vi "GET_sendStatusToClient.vi"() -> (0 "position":dbl, 1 "mode":string)   [LabVIEW 2024]
uses:
  <vilib>/wsapi/Web Request.lvclass
  Main.vi
panel:
  in  "LabVIEW Web Service Request":refnum<class "Web Request.lvclass">
  # "Use the Web Service Request input terminal to call the VIs on the Web Services palette. Do not remove it from the connector pane unless you don't need access to the palette."
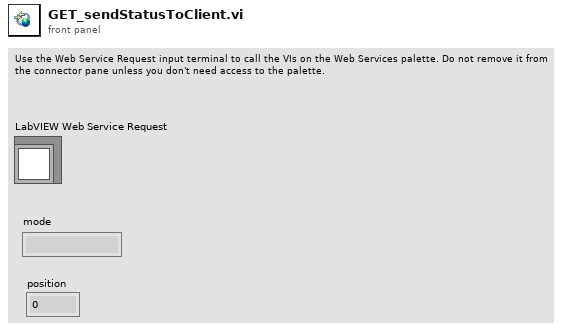
[diagram p1: front panel]
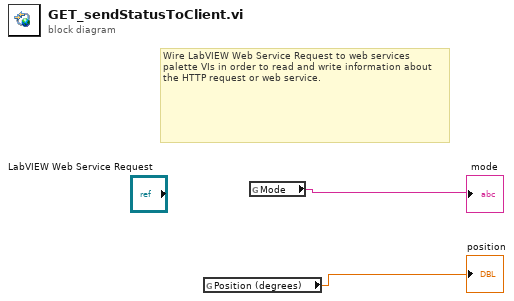
[diagram p0: block diagram]
diagram:
  # "Wire LabVIEW Web Service Request to web services palette VIs in order to read and write information about the HTTP request or web service."
  n1 = global read "Main.vi" "Position (degrees)"() -> (→"position":dbl)
  n2 = global read "Main.vi" "Mode"() -> (→"mode":string)
